vi "Destroy.vi"(8 "Error In":errorcluster, 11 "object in":refnum<class "Component.Tabulator.lvclass">) -> (0 "Error Out":errorcluster)   [LabVIEW 2020, in "Component.Tabulator.lvclass"]
uses:
  Component.Tabulator.lvclass
  Component_class/Component.lvclass
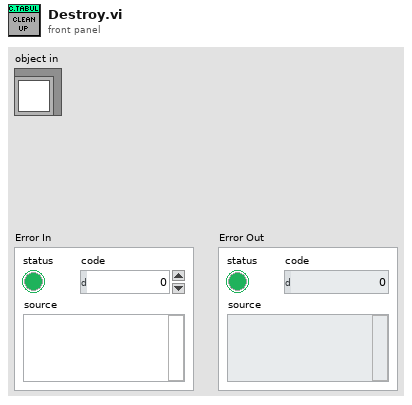
[diagram p1: front panel]
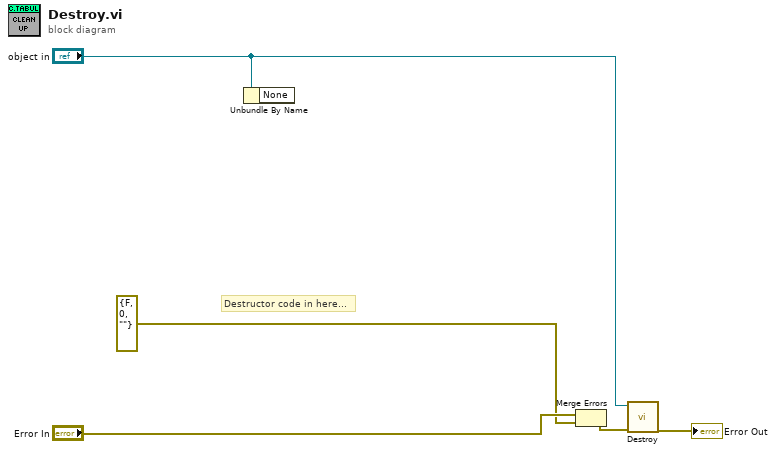
[diagram p0: block diagram]
diagram:
  # "Destructor code in here..."
  n1 = Unbundle By Name("object in") -> ()  [unwired: 1 out]
  n2 = Merge Errors("Error In", errorcluster {"status"=FALSE, "code"=0, "source"=""} ("error in (no error)")) -> (w2:errorcluster)
  n3 = call-parent "Destroy.vi"("Error In"=w2, "object in"="object in") -> ("Error Out"=→"Error Out":errorcluster)  [unwired: 9 in]
